vi "Init AI DAQ.vi"(0 "DaqDevice":string="PCI6232", 1 "number samples":i32=1000, 3 "LoadCellParams":T2={"Excitation Value (Volts)"=2.5, "mV/V"=2.0, "Max Weight (lbs)"=500.0}, 5 "Physical Channels":string[](array[string])=["ai0", "ai1"], 9 "Type":enum16{"Voltage", "Current", "LoadCell"}(ring), 11 "error in":errorcluster, 12 "Rate":dbl=25000.0, 13 "PerformNullOffset":bool, 14 "ShuntCalParams":T1={"Load Cell bridge resistance (Ohms)"=120.0, "9237 Internal shunt resistance (Ohms)"=100000.0, "shunt element location"=14813} {"shunt element location" items=["R1"=12465, "R2"=12466, "R3"=12467, "R4"=14813, "None"=10230]; "9237 Internal shunt resistance (Ohms)" format="%#.3p"}) -> (4 "task out":refnum<k21>, 15 "error out":errorcluster)   [LabVIEW 2017]
doc: "Developed by Kevin Thompson\nThompson Engineering, LLC\nkevin@thompsonengineering.net"
uses:
  <vilib>/DAQmx/create/channels.llb/DAQmx Create Channel (AI-Voltage-Basic).vi
  <vilib>/DAQmx/create/channels.llb/DAQmx Create Channel (AI-Current-Basic).vi
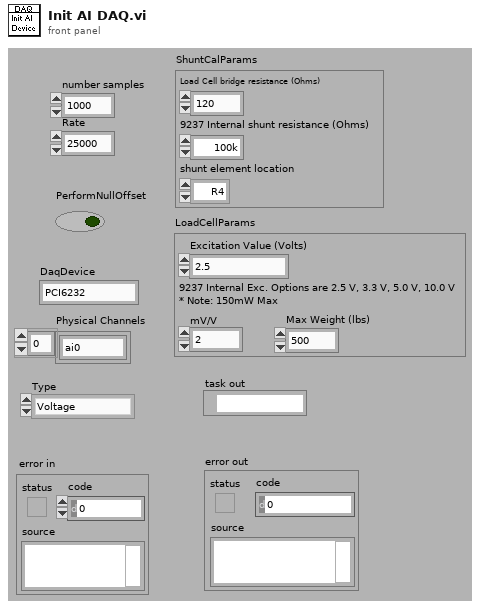
[diagram p1: front panel]
types:
  T1 = cluster{"Load Cell bridge resistance (Ohms)":dbl, "9237 Internal shunt resistance (Ohms)":dbl, "shunt element location":i32}
  T2 = cluster{"Excitation Value (Volts)":dbl, "mV/V":dbl, "Max Weight (lbs)":dbl}
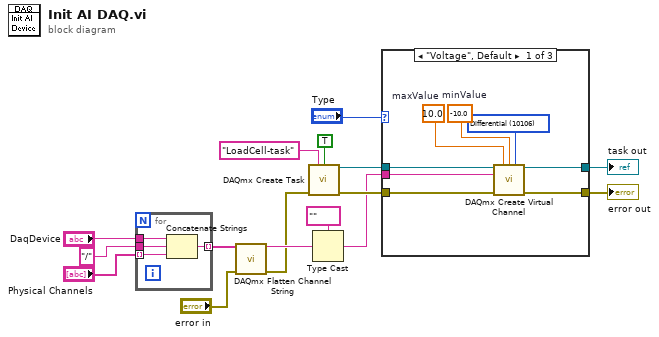
[diagram p0: block diagram]
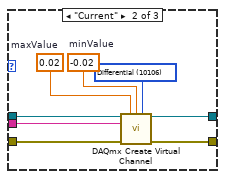
[diagram p2: hidden frame]
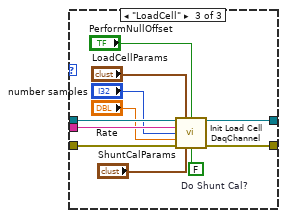
[diagram p3: hidden frame]
diagram:
  n1 = for {
    tunnel: "/" -> [w20]
    tunnel: "DaqDevice" -> [w19]
    tunnel: "Physical Channels" -> [w18] mode=indexing
    tunnel: [w17] -> w7 mode=indexing
    n2 = Concatenate Strings(w19, w20, w18) -> (w17:string)
  }
  n3 = call <vilib>:"DAQmx Flatten Channel String.vi"("names in"=w7, "error in"="error in") -> ("names out"=w6:string, "error out"=w3:errorcluster)  [unwired: 12 in]
  n4 = call <vilib>:"DAQmx Create Task.vi"("new task name"="LoadCell-task", "auto cleanup"=TRUE, "error in"=w3) -> ("task out"=w14:refnum<k21>, "error out"=w11:errorcluster)  [unwired: 11 in]
  n5 = Type Cast(type=tag "" ("PhysChan"), x=w6) -> (*(type *) &x=w5:tag)
  n6 = case shown="\"Voltage\", Default" "Type" {
    tunnel: w14 -> [w28 w36 w47]
    tunnel: w5 -> [w27 w35 w46]
    tunnel: w11 -> [w23 w31 w45]
    tunnel: [w22 w30 w44] -> w10
    tunnel: [w21 w29 w43] -> w2
    frame "Voltage", Default {
      w24 = 10.0  # maxValue
      w25 = -10.0  # minValue
      w26 = 10106 items=["default"=-1, "RSE"=10083, "NRSE"=10078, "Differential"=10106, "Pseudodifferential"=12529] ("termConfig")
      n7 = call-poly <vilib>:"DAQmx Create Virtual Channel.vi"("task in"=w28, "maximum value"=w24, "minimum value"=w25, "input terminal configuration"=w26, "physical channels"=w27, "error in"=w23) -> ("task out"=w21:refnum<k21>, "error out"=w22:errorcluster)  [unwired: 8 in]
    }
    frame "Current" {
      w32 = 0.02  # maxValue
      w33 = -0.02  # minValue
      w34 = 10106 items=["default"=-1, "RSE"=10083, "NRSE"=10078, "Differential"=10106, "Pseudodifferential"=12529] ("termConfig")
      n8 = call-poly <vilib>:"DAQmx Create Virtual Channel.vi"("task in"=w36, "maximum value"=w32, "minimum value"=w33, "input terminal configuration"=w34, "physical channels"=w35, "error in"=w31) -> ("task out"=w29:refnum<k21>, "error out"=w30:errorcluster)  [unwired: 8 in]
    }
    frame "LoadCell" {
      w38 = FALSE  # Do Shunt Cal?
      n9 = call "Init Load Cell DaqChannel.vi"("task in"=w47, "LoadCellParams"="LoadCellParams", "Do Offset Null?"="PerformNullOffset", "Physical Channels"=w46, "number samples"="number samples", "Rate"="Rate", "error in (no error)"=w45, "ShuntCalParams"="ShuntCalParams", "Do Shunt Cal?"=w38) -> ("task out"=w43:refnum<k21>, "error out"=w44:errorcluster)  [unwired: 5 in]
    }
  }
  "task out" <- w2
  "error out" <- w10
